vi "YAV IOPSx.vi"() -> ()   [LabVIEW 2018]
uses:
  <instrlib>/Phi6/Common/Instrum/Phi6 Core/YAV-System.llb/YAV Card Total Info.ctl
  <instrlib>/Phi6/Common/Instrum/Phi6 Core/YAV-System.llb/YAV Info.ctl
  <instrlib>/Phi6/Common/Instrum/Phi6 Core/YAV-90132.llb/YAV90132 Type Action.ctl
  <instrlib>/Phi6/Common/Instrum/Phi6 Core/YAV-90132.llb/YAV90132 Mode Action.ctl
  <instrlib>/Phi6/Common/Instrum/Phi6 Core/CANNOU Global Variables.llb/CANNOU Global Variables.gbl.vi
panel:
  in  "Average":u32
  in  "Info In":T1 {"Version" format="%.0x"; "Options" format="%.0x"; "Index" format="%.0x"}
  out "IOPS":u32
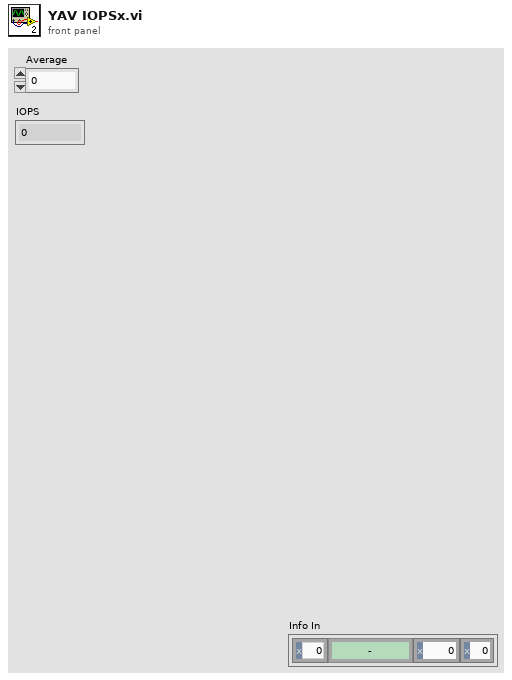
[diagram p1: front panel]
types:
  T1 = typedef "YAV Card Total Info.ctl" = cluster{"Index":u8, "Module":T2, "Version":u16, "Options":u8}
  T2 = typedef "YAV Info.ctl" = enum16{"-", "YAV90832", "YAV904X8", "YAV90132", "YAV91616", "YAV90PIN", "YAV90096", "YAV90HVT", "YAV90CLR", "YAV90128", "YAV90PNE", "YAVCANCON", "YAV91775", "YAV90XXX", "YAV90MMU", "H730050", "H710060", "H710061", "YAV90304", "MMI", "YAV90060", "YAV90MUX", "YAV90059", "YAV90070", "AK087", "Not Defined"}
  T3 = typedef "YAV90132 Type Action.ctl" = enum16{"None", "Set OFF", "Set ON", "TOGGLE", "BLINK", "PULSE ON", "PULSE OFF", "ASK", "Set OUT"}
  T4 = typedef "YAV90132 Mode Action.ctl" = enum16{"None", "One Relay", "Several Relays"}
  T5 = typedef "Module CAN.ctl" = enum16{"CAN0", "CAN1", "CAN2", "CAN3", "CAN4", "CAN5"}
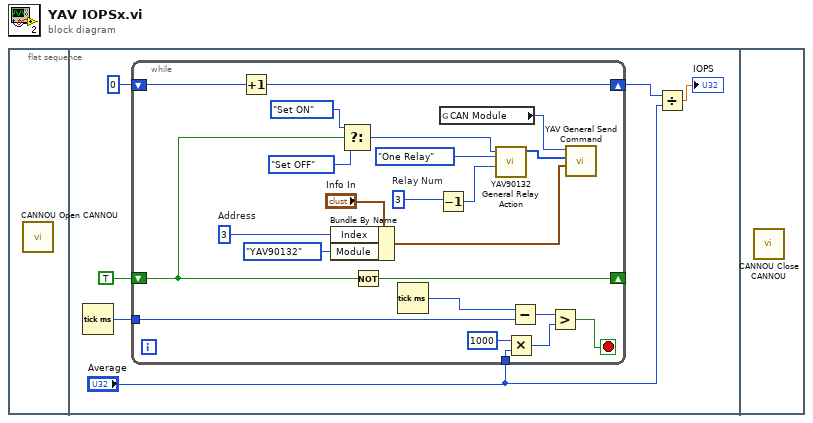
[diagram p0: block diagram]
diagram:
  n1 = flat-sequence {
    frame #0 {
      n2 = call <instrlib>:"CANNOU Open CANNOU.vi"() -> ()  [unwired: 6 in, 2 out]
    }
    frame #1 {
      n3 = Tick Count (ms)() -> (millisecond timer value=w6:u32)
      n4 = while {
        tunnel: w6 -> [w28]
        shift-right: [w25] -> w3
        shift-left: u32 0 ("x") -> [w26]
        shift-right: [w23] -> _
        shift-left: TRUE ("State") -> [w10]
        tunnel: "Average" -> [w7]
        stop <- w27 stop-if-true
        w15 = u8 3  # Address
        w16 = u32 3  # Relay Num
        n5 = Increment(x=w26) -> (x+1=w25:u32)
        n6 = Bundle By Name(cluster="Info In", "Index"=w15, "Module"=YAV_Info."YAV90132") -> (w21:T1)
        n7 = Select(t=YAV90132_Type_Action."Set ON" ("Type Action"), s=w10, f=YAV90132_Type_Action."Set OFF") -> (s? t:f=w19:T3)
        n8 = Not(x=w10) -> (.not. x?=w23:bool)
        n9 = Tick Count (ms)() -> (millisecond timer value=w29:u32)
        n10 = Decrement(x=w16) -> (x-1=w22:u32)
        n11 = global read "CANNOU Global Variables.gbl.vi" "CAN Module"() -> (w18:T5)
        n12 = call <instrlib>:"YAV90132 General Relay Action.vi"("Relay/Relays"=w22, "Mode Action"=YAV90132_Mode_Action."One Relay", "Type Action"=w19) -> ("Data"=w20:u8[])  [unwired: 8 in]
        n13 = Multiply(x=u32 1000, y=w7) -> (x*y=w8:u32)
        n14 = Subtract(x=w29, y=w28) -> (x-y=w24:u32)
        n15 = Greater?(x=w24, y=w8) -> (0:w27:bool)
        n16 = call <instrlib>:"YAV General Send Command.vi"("Info In"=w21, "Data"=w20, "CAN Module"=w18) -> ()  [unwired: 3 in, 2 out]
      }
      n17 = Divide(x=w3, y="Average") -> (x/y=→"IOPS":dbl)
    }
    frame #2 {
      n18 = call <instrlib>:"CANNOU Close CANNOU.vi"() -> ()  [unwired: 7 in, 1 out]
    }
  }
